vi "Rename.vi"() -> ()   [LabVIEW 2020]
uses:
  _Rename/_Rename/_Rename.lvclass
  _Shared/_Shared.lvlib
  _Shared/Tree/Tree.lvlib
  _Shared/Name Specs/Name Specs.lvclass
panel:
  out "Target":string
  in  "Tree":string(tree)
  in  "OK":bool
  in  "Rename":string
  # "Disclaimer: Please consider committing changes before AND after this action."
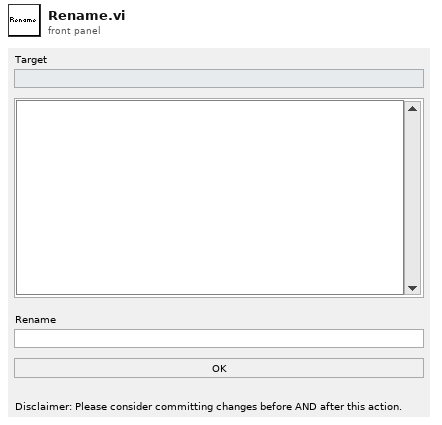
[diagram p1: front panel]
types:
  T1 = enum32{"Invalid", "Standard", "Closed", "Hidden", "Minimized", "Maximized"}
  T2 = typedef "_Shared.lvlib/Type Name Library File Path.ctl" = map{T3, T4}
  T3 = typedef "_Shared.lvlib/Type.ctl" = enum16{"Actor", "Msg"}
  T4 = typedef "_Shared.lvlib/Name Library File Path.ctl" = map{string, path}
  T5 = typedef "_Shared.lvlib/Name Stuff.ctl" = cluster{"Type (Enum)":T3, "Type (String)":string, "Name Library File Path":path, "Name":string, "Name Type":string}
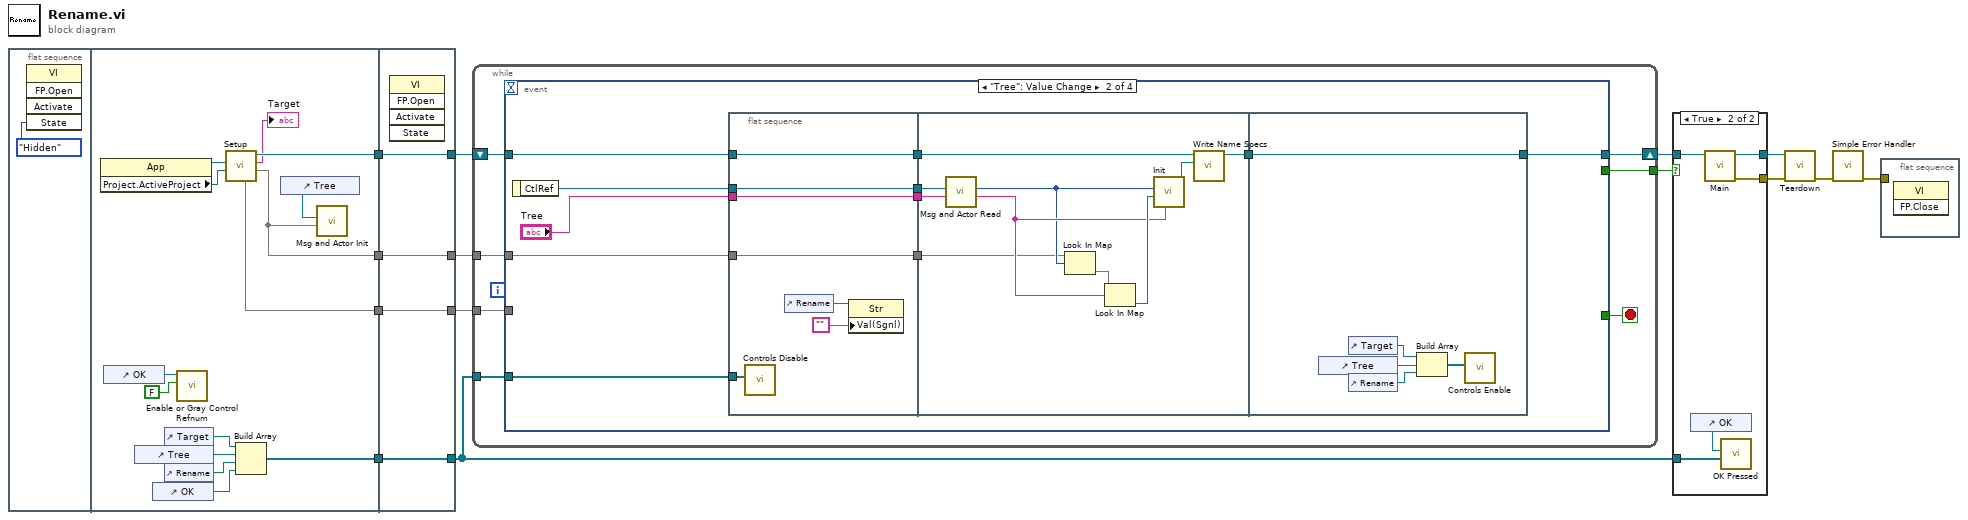
[diagram p0: block diagram]
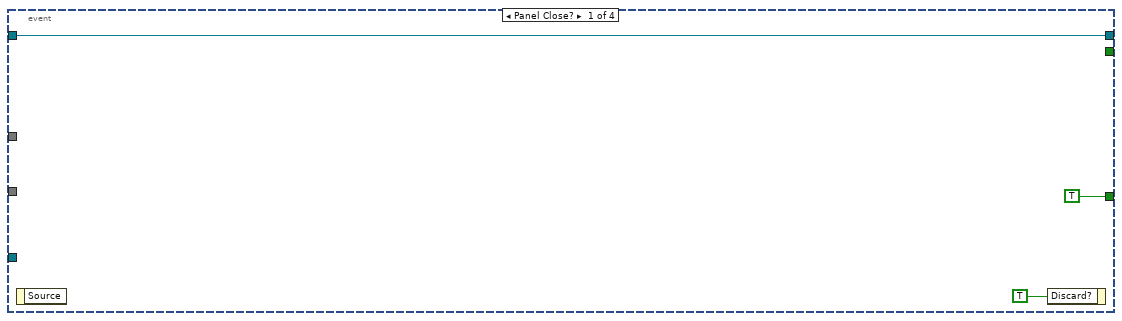
[diagram p2: hidden frame]
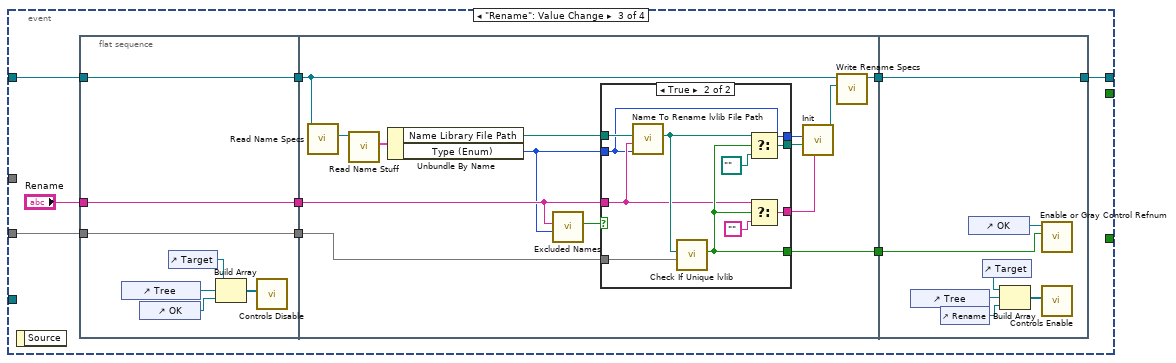
[diagram p3: hidden frame]
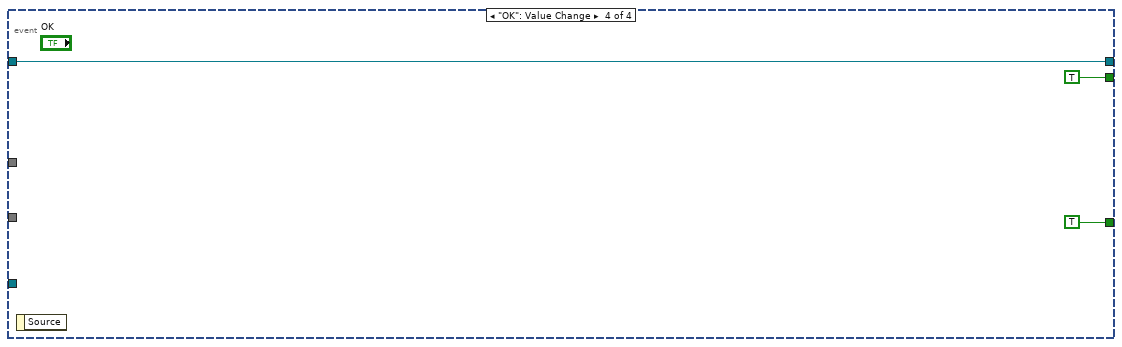
[diagram p5: hidden frame]
diagram:
  n1 = flat-sequence {
    tunnel: [w17] -> w9
    tunnel: [w26] -> w7
    tunnel: [w22] -> w6
    tunnel: [w16] -> w1
    tunnel: [w33] -> w10
    tunnel: w9 -> [w33]
    tunnel: [w32] -> w8
    tunnel: w7 -> [w32]
    tunnel: [w31] -> w5
    tunnel: w6 -> [w31]
    tunnel: [w30] -> w2
    tunnel: w1 -> [w30]
    frame #0 {
      n2 = invoke class="VI" method="FP.Open"("State"=T1."Hidden") -> ()  [unwired: 4 in, 5 out]
    }
    frame #1 {
      n3 = property class="App"() -> (reference out=w27:refnum<vi>, "Project.ActiveProject"=w28:refnum<vi>)  [unwired: 2 in, 1 out]
      n4 = control-ref of="OK"() -> (w21:refnum<vi>)
      n5 = control-ref of="Tree"() -> (w25:refnum<vi>)
      n6 = control-ref of="OK"() -> (w23:refnum<vi>)
      n7 = control-ref of="Target"() -> (w18:refnum<vi>)
      n8 = control-ref of="Rename"() -> (w24:refnum<vi>)
      n9 = call <vilib>:"Enable or Gray Control Refnum.vi"("enable?"=FALSE, "Control in"=w21) -> ()  [unwired: 8 in, 2 out]
      n10 = call "Setup.vi"("Active Project"=w28, "NI.LV.Dialog Instance"=w27) -> ("Project Type Name Library File Path"=w16:T2, "Target"=→"Target":string, "Script out"=w26:refnum<class "_Rename.lvclass">, "All Type Name Library File Path"=w17:T2)  [unwired: 6 in]
      n11 = Build Array(w18, w25, w24, w23) -> (w22:refnum<vi>[])
      n12 = control-ref of="Tree"() -> (w29:refnum<vi>)
      n13 = call "Msg and Actor Init.vi"("Type Name Library File Path"=w16, "Tree Ref"=w29) -> ()  [unwired: 10 in]
    }
    frame #2 {
      n14 = invoke class="VI" method="FP.Open"() -> ()  [unwired: 5 in, 5 out]
    }
  }
  n15 = while {
    tunnel: [w40] -> w12
    shift-right: [w37] -> w11
    shift-left: w8 -> [w38]
    tunnel: w10 -> [w36]
    tunnel: w5 -> [w35]
    tunnel: w2 -> [w34]
    stop <- w39 stop-if-true
    n16 = event shown="[1] \"Tree\": Value Change" {
      selector: _ -> [_ _ _ _]
      dyn-events: _ -> [_ _ _ _]
      timeout: _ -> [_ _ _ _]
      tunnel: [_ _ _ TRUE ("Rename 2")] -> w40
      tunnel: [TRUE _ _ TRUE] -> w39
      tunnel: w38 -> [w41 w52 w82 w124]
      tunnel: [w41 w54 w85 w124] -> w37
      tunnel: w36 -> [_ _ w81 _]
      tunnel: w35 -> [_ w46 _ _]
      tunnel: w34 -> [_ w44 _ _]
      event Panel Close? {
        n17 = event-data() -> ()  [unwired: 1 in, 1 out]
        n18 = event-data("Discard?"=TRUE) -> ()  [unwired: 1 in, 1 out]
      }
      event "Tree": Value Change {
        n19 = event-data() -> ("CtlRef"=w50:refnum<vi>)  [unwired: 1 in]
        n20 = flat-sequence {
          tunnel: w50 -> [w59]
          tunnel: "Tree" -> [w60]
          tunnel: w52 -> [w61]
          tunnel: [w61] -> w49
          tunnel: [w60] -> w48
          tunnel: [w59] -> w47
          tunnel: w46 -> [w58]
          tunnel: [w55] -> w45
          tunnel: w44 -> [w55]
          tunnel: [w64] -> w53
          tunnel: w49 -> [w65]
          tunnel: w48 -> [w70]
          tunnel: w47 -> [w69]
          tunnel: w45 -> [w62]
          tunnel: [w73] -> w54
          tunnel: w53 -> [w73]
          frame #0 {
            n21 = call "Controls Disable.vi"("Controls in"=w58) -> ()  [unwired: 11 in]
            n22 = control-ref of="Rename"() -> (w57:refnum<vi>)
            n23 = property class="Str"(reference=w57, "Val(Sgnl)"="") -> ()  [unwired: 1 in, 2 out]
          }
          frame #1 {
            n24 = call "Msg and Actor Read.vi"("Tree"=w70, "Tree Ref"=w69) -> ("Name"=w66:string, "Type"=w63:T3)  [unwired: 8 in]
            n25 = Look In Map(map=w62, key=w63) -> (value=w71:T4)  [unwired: 1 in, 1 out]
            n26 = Look In Map(map=w71, key=w66) -> (value=w67:path)  [unwired: 1 in, 1 out]
            n27 = call "Init.vi"("Name"=w66, "Name Library File Path"=w67, "Type"=w63) -> ("Name Specs out"=w68:refnum<class "Name Specs.lvclass">)  [unwired: 8 in]
            n28 = call "Write Name Specs.vi"("Name Specs"=w68, "_Rename in"=w65) -> ("_Rename out"=w64:refnum<class "_Rename.lvclass">)  [unwired: 9 in]
          }
          frame #2 {
            n29 = control-ref of="Tree"() -> (w75:refnum<vi>)
            n30 = control-ref of="Target"() -> (w72:refnum<vi>)
            n31 = control-ref of="Rename"() -> (w76:refnum<vi>)
            n32 = Build Array(w72, w75, w76) -> (w74:refnum<vi>[])
            n33 = call "Controls Enable.vi"("Controls in"=w74) -> ()  [unwired: 11 in]
          }
        }
      }
      event "Rename": Value Change {
        n34 = event-data() -> ()  [unwired: 1 in, 1 out]
        n35 = flat-sequence {
          tunnel: "Rename" -> [w90]
          tunnel: w81 -> [w91]
          tunnel: w82 -> [w92]
          tunnel: [w92] -> w79
          tunnel: [w91] -> w78
          tunnel: [w90] -> w77
          tunnel: [w105] -> w84
          tunnel: [w98] -> w83
          tunnel: w79 -> [w97]
          tunnel: w78 -> [w106]
          tunnel: w77 -> [w94]
          tunnel: [w118] -> w85
          tunnel: w84 -> [w119]
          tunnel: w83 -> [w118]
          frame #0 {
            n36 = control-ref of="Tree"() -> (w87:refnum<vi>)
            n37 = control-ref of="OK"() -> (w88:refnum<vi>)
            n38 = control-ref of="Target"() -> (w86:refnum<vi>)
            n39 = Build Array(w86, w87, w88) -> (w89:refnum<vi>[])
            n40 = call "Controls Disable.vi"("Controls in"=w89) -> ()  [unwired: 11 in]
          }
          frame #1 {
            n41 = call "Read Name Specs.vi"("_Rename in"=w97) -> ("Name Specs"=w104:refnum<class "Name Specs.lvclass">)  [unwired: 10 in]
            n42 = call "Read Name Stuff.vi"("Name Specs in"=w104) -> ("Name Stuff"=w103:T5)  [unwired: 10 in]
            n43 = Unbundle By Name(w103) -> ("Name Library File Path"=w102:path, "Type (Enum)"=w93:T3)
            n44 = call "Excluded Names.vi"("Type"=w93, "Rename"=w94) -> ("Valid"=w95:bool)  [unwired: 9 in]
            n45 = case shown="True" w95 {
              tunnel: [_ w114] -> w105
              tunnel: w106 -> [_ w109]
              tunnel: w94 -> [_ w108]
              tunnel: [_ w111] -> w99
              tunnel: [_ w116] -> w100
              tunnel: w102 -> [_ w115]
              tunnel: w93 -> [_ w107]
              tunnel: [_ w107] -> w96
              frame False {
              }
              frame True {
                n46 = call "Name To Rename lvlib File Path.vi"("Type"=w107, "Rename"=w108, "Name Library File Path"=w115) -> ("Rename Library File Path"=w113:path)  [unwired: 8 in]
                n47 = call "Check If Unique lvlib.vi"("All Type Name Library File Path"=w109, "Library File Path"=w113) -> ("Unique?"=w114:bool)  [unwired: 9 in]
                n48 = Select(t=w113, s=w114, f=path "") -> (s? t:f=w111:path)
                n49 = Select(t=w108, s=w114, f="") -> (s? t:f=w116:string)
              }
            }
            n50 = call "Init.vi"("Name"=w100, "Name Library File Path"=w99, "Type"=w96) -> ("Name Specs out"=w101:refnum<class "Name Specs.lvclass">)  [unwired: 8 in]
            n51 = call "Write Rename Specs.vi"("Rename Specs"=w101, "_Rename in"=w97) -> ("_Rename out"=w98:refnum<class "_Rename.lvclass">)  [unwired: 9 in]
          }
          frame #2 {
            n52 = control-ref of="Tree"() -> (w123:refnum<vi>)
            n53 = control-ref of="Rename"() -> (w121:refnum<vi>)
            n54 = control-ref of="OK"() -> (w120:refnum<vi>)
            n55 = control-ref of="Target"() -> (w117:refnum<vi>)
            n56 = Build Array(w117, w123, w121) -> (w122:refnum<vi>[])
            n57 = call <vilib>:"Enable or Gray Control Refnum.vi"("enable?"=w119, "Control in"=w120) -> ()  [unwired: 8 in, 2 out]
            n58 = call "Controls Enable.vi"("Controls in"=w122) -> ()  [unwired: 11 in]
          }
        }
      }
      event "OK": Value Change {
        n59 = event-data() -> ()  [unwired: 1 in, 1 out]
      }
    }
  }
  n60 = case shown="True" w12 {
    tunnel: w11 -> [w127 w132]
    tunnel: [w127 w131] -> w14
    tunnel: w5 -> [_ w128]
    tunnel: [_ w130] -> w13
    frame False {
    }
    frame True {
      n61 = control-ref of="OK"() -> (w129:refnum<vi>)
      n62 = call "Main.vi"("_Rename in"=w132) -> ("error out"=w130:errorcluster, "_Rename out"=w131:refnum<class "_Rename.lvclass">)  [unwired: 9 in]
      n63 = call "OK Pressed.vi"("Controls in"=w128, "OK Ref"=w129) -> ()  [unwired: 10 in]
    }
  }
  n64 = call "Teardown.vi"("error in"=w13, "_Rename in"=w14) -> ("error out"=w4:errorcluster)  [unwired: 9 in]
  n65 = call <vilib>:"Simple Error Handler.vi"("error in (no error)"=w4) -> ("error out"=w3:errorcluster)  [unwired: 4 in, 4 out]
  n66 = flat-sequence {
    tunnel: w3 -> [_]
    frame #0 {
      n67 = invoke class="VI" method="FP.Close"() -> ()  [unwired: 3 in, 3 out]
    }
  }
